vi "close.vi"(8 "error in (no error)":errorcluster, 11 "CameraNetworkController in":refnum<class "CameraNetworkController.lvclass">) -> (0 "error out":errorcluster, 3 "CameraNetworkController out":refnum<class "CameraNetworkController.lvclass">)   [LabVIEW 2011, in "Hardware.lvlib" / "HWControllers.lvlib" / "CameraNetworkController.lvclass"]
uses:
  CameraNetworkController.lvclass
  NetworkClient/NetworkServer.lvclass
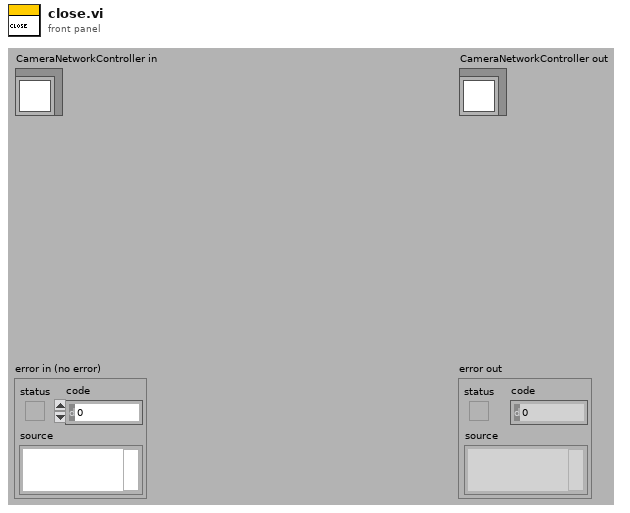
[diagram p1: front panel]
types:
  T1 = cluster{"Message":enum16{"Idle", "initialise", "configureAcquisition", "setTemperature", "getTemperature", "start", "stop", "sendImage", "close", "error", "ExitApp"}, "Data":variant}
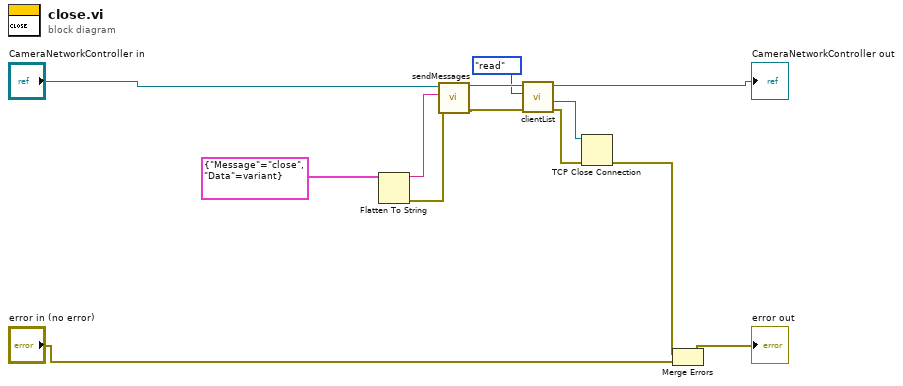
[diagram p0: block diagram]
diagram:
  n1 = Flatten To String(anything=T1 {"Message"=enum."close", "Data"=variant}) -> (data string=w11:string, error out=w12:errorcluster)  [unwired: 1 in, 3 out]
  n2 = call "sendMessages.vi"("error in (no error)"=w12, "messageString"=w11, "NetworkClient in"="CameraNetworkController in") -> ("error out"=w5:errorcluster, "NetworkClient out"=w7:refnum<class "CameraNetworkController.lvclass">)  [unwired: 7 in]
  n3 = call "clientList.vi"("error in (no error)"=w5, "Enum"=enum16{"read", "write", "reset"}."read", "NetworkServer in"=w7) -> ("error out"=w4:errorcluster, "client"=w3:refnum<k5>, "NetworkServer out"=→"CameraNetworkController out":refnum<class "CameraNetworkController.lvclass">)  [unwired: 5 in, 1 out]
  n4 = TCP Close Connection(connection ID=w3, error in (no error)=w4) -> (error out=w2:errorcluster)  [unwired: 1 in, 1 out]
  n5 = Merge Errors(w2, "error in (no error)") -> (→"error out":errorcluster)
